vi "data insert core.vi"(8 "error in (no error)":errorcluster, 9 "column information":T1[](array[typedef]), 10 "data":variant[](array[variant]), 11 "table":string) -> (0 "error out":errorcluster)   [LabVIEW 2016, in "质控单元.lvlib"]
uses:
  <vilib>/addons/database/Auxilliary.llb/DB Tools Column Info.ctl
  <vilib>/addons/database/Auxilliary.llb/DB Tools DataTypes.ctl
  <vilib>/addons/database/Auxilliary.llb/DB Tools Transaction.ctl
  <vilib>/addons/database/Auxilliary.llb/DB Tools Isolation Level.ctl
  <vilib>/Utility/sysdir.llb/System Directory Type.ctl
  <vilib>/addons/database/Auxilliary.llb/DB Tools Parameter Info.ctl
  <vilib>/addons/database/Auxilliary.llb/DB Tools Parameter Dir.ctl
  <vilib>/addons/database/Connection.llb/DB Tools Open Connec (String).vi
  <vilib>/addons/database/Connection.llb/Conn Transaction.vi
  <vilib>/addons/database/Connection.llb/Conn Execute.vi
  <vilib>/addons/database/Recordset.llb/Rec Destroy - Connection.vi
  <vilib>/addons/database/Command.llb/Cmd Set Parameter Value (C).vi
  <vilib>/addons/database/Auxilliary.llb/DB Tools Format Datetime String (Time Stamp).vi
  <vilib>/addons/database/Command.llb/Cmd Execute.vi
  <vilib>/addons/database/Recordset.llb/Rec Destroy - Command.vi
  <vilib>/addons/database/Command.llb/Cmd Delete.vi
  <vilib>/addons/database/NI_Database_API.lvlib
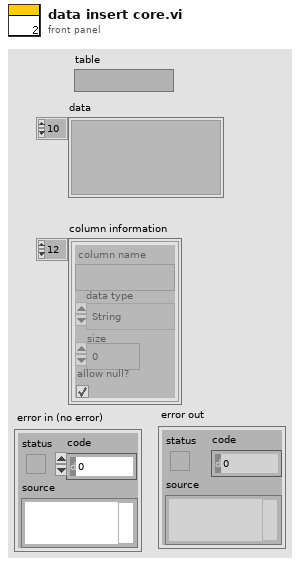
[diagram p1: front panel]
types:
  T1 = typedef "NI_Database_API.lvlib/DB Tools Column Info.ctl" = cluster{"column name":string, "data type":T2, "size":i32, "allow null?":bool}
  T2 = typedef "NI_Database_API.lvlib/DB Tools DataTypes.ctl" = enum16{"String", "Long (I32)", "Single (SGL)", "Double (DBL)", "Date/Time", "Binary"}
  T3 = typedef "System Directory Type.ctl" = i32
  T4 = typedef "NI_Database_API.lvlib/DB Tools Isolation Level.ctl" = enum16{"chaos", "read uncommitted", "read committed", "repeatable read", "serializable"}
  T5 = typedef "NI_Database_API.lvlib/DB Tools Transaction.ctl" = enum16{"begin", "commit", "rollback"}
  T6 = typedef "NI_Database_API.lvlib/Conn ObjectReference.ctl" = refnum<k1>
  T7 = typedef "NI_Database_API.lvlib/DB Tools Parameter Info.ctl" = cluster{"parameter name":string, "type":T2, "direction":T8, "value":variant}
  T8 = typedef "NI_Database_API.lvlib/DB Tools Parameter Dir.ctl" = enum32{"Input", "Output", "Input/Output", "Return Value"}
  T9 = typedef "NI_Database_API.lvlib/Rec ObjectReference.ctl" = refnum<k1>
  T10 = typedef "NI_Database_API.lvlib/Cmd ObjectReference.ctl" = refnum<k1>
  T11 = typedef "NI_Database_API.lvlib/Cmd-Rec Object Reference.ctl" = refnum<k1>
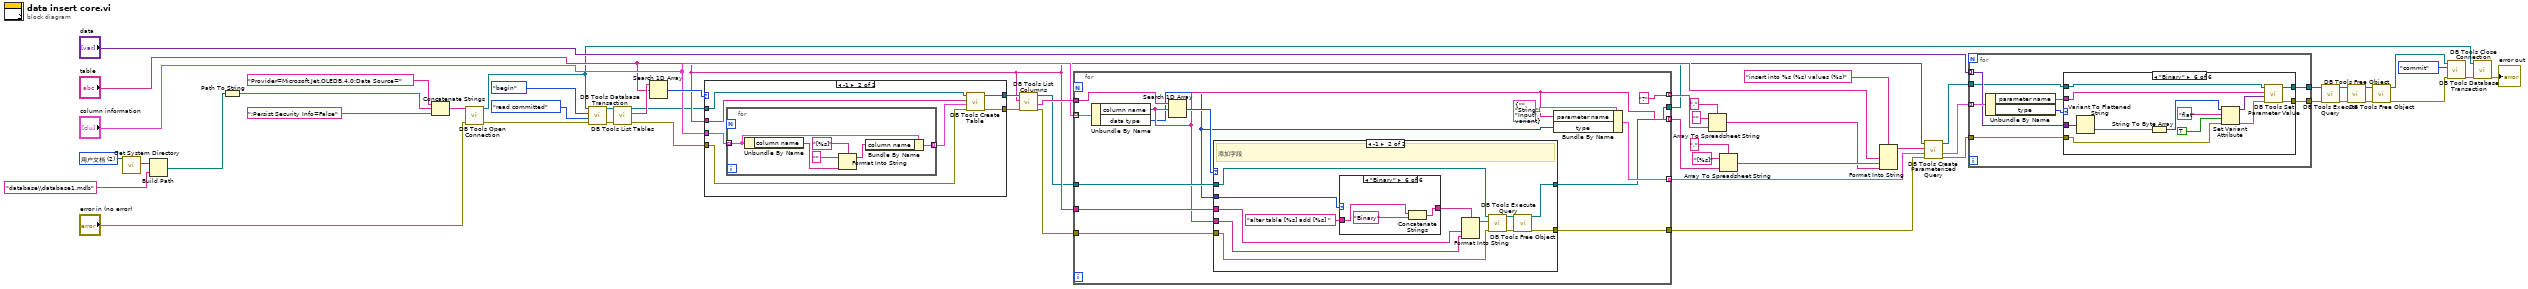
[diagram p0: block diagram]
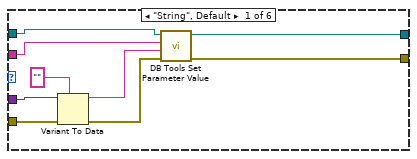
[diagram p2: hidden frame]
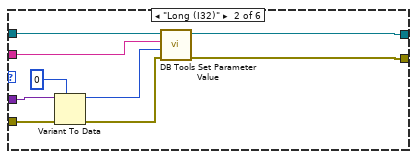
[diagram p3: hidden frame]
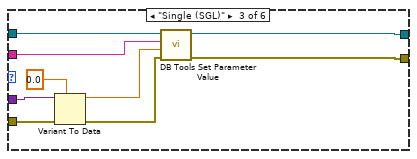
[diagram p4: hidden frame]
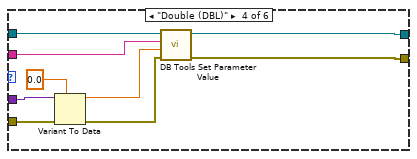
[diagram p5: hidden frame]
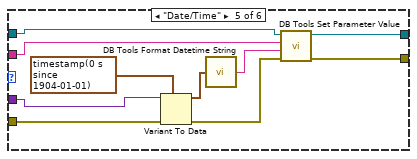
[diagram p6: hidden frame]
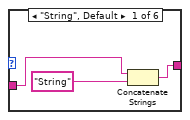
[diagram p8: hidden frame]
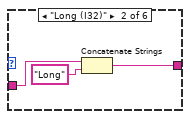
[diagram p9: hidden frame]
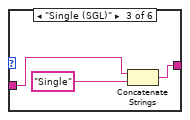
[diagram p10: hidden frame]
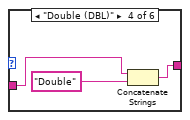
[diagram p11: hidden frame]
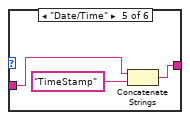
[diagram p12: hidden frame]
diagram:
  w3 = T3 2 items=["用户目录"=0, "用户桌面"=1, "用户文档"=2, "用户应用程序数据"=3, "用户设置"=4, "用户临时目录"=5, "公共文档"=6, "公共应用程序数据"=7, "公共设置"=8, "公共缓存"=13, "系统核心库"=9, "系统安装库"=10, "应用程序文件"=11, "启动盘根目录"=12] ("system directory type")
  n1 = call <vilib>:"Get System Directory.vi"("system directory type"=w3) -> ("system directory"=w4:path)  [unwired: 10 in]
  n2 = Build Path(base path=w4, name or relative path="database\\database1.mdb" ("名称或相对路径")) -> (appended path=w2:path)
  n3 = Path To String(path=w2) -> (string=w53:string)
  n4 = Concatenate Strings("Provider=Microsoft.Jet.OLEDB.4.0;Data Source=" ("condition"), w53, ";Persist Security Info=False" ("condition")) -> (w51:string)
  n5 = call-poly <vilib>:"DB Tools Open Connection.vi"("error in (no error)"="error in (no error)", "connection information"=w51) -> ("error out"=w13:errorcluster, "connection reference"=w5:T6)  [unwired: 6 in]
  n6 = call-poly <vilib>:"DB Tools Database Transaction.vi"("error in (no error)"=w13, "isolation level (chaos)"=DB_Tools_Isolation_Level."read committed", "operation (begin)"=DB_Tools_Transaction."begin", "connection reference"=w5) -> ("error out"=w12:errorcluster, "connection reference out"=w14:T6)  [unwired: 2 in]
  n7 = call <vilib>:"DB Tools List Tables.vi"("error in (no error)"=w12, "connection reference"=w14) -> ("error out"=w43:errorcluster, "tables"=w45:string[], "connection reference out"=w8:T6)  [unwired: 3 in]
  n8 = Search 1D Array(1D array=w45, element="table") -> (index of element=w44:i32)  [unwired: 1 in]
  n9 = case shown="-1" w44 {
    tunnel: w8 -> [w56 w63]
    tunnel: w43 -> [w55 w62]
    tunnel: "table" -> [_ w61]
    tunnel: "column information" -> [_ w58]
    tunnel: [w56 w60] -> w39
    tunnel: [w55 w59] -> w38
    frame 0, Default {
    }
    frame -1 {
      n10 = for {
        tunnel: w58 -> [w65] mode=indexing
        tunnel: [w64] -> w57 mode=indexing
        n11 = Unbundle By Name(w65) -> ("column name"=w69:string)
        n12 = Format Into String(format string="[%s]" ("格式字符串"), initial string="" ("初始字符串"), w69) -> (resulting string=w66:string)  [unwired: 1 in, 1 out]
        n13 = Bundle By Name(cluster=w65, "column name"=w66) -> (w64:T1)
      }
      n14 = call <vilib>:"DB Tools Create Table.vi"("error in (no error)"=w62, "column information"=w57, "table"=w61, "connection reference"=w63) -> ("error out"=w59:errorcluster, "connection reference out"=w60:T6)  [unwired: 4 in]
    }
  }
  n15 = call <vilib>:"DB Tools List Columns.vi"("error in (no error)"=w38, "table"="table", "connection reference"=w39) -> ("error out"=w41:errorcluster, "columns"=w42:string[], "connection reference out"=w10:T6)  [unwired: 1 in, 1 out]
  n16 = for {
    tunnel: w10 -> [w80]
    tunnel: w42 -> [w82]
    tunnel: w41 -> [w79]
    tunnel: [w78] -> w37
    tunnel: "table" -> [w77]
    tunnel: "column information" -> [w76] mode=indexing
    tunnel: [w74] -> w36 mode=indexing
    tunnel: [w73] -> w29 mode=indexing
    tunnel: ["?"] -> w27 mode=indexing
    tunnel: [w70] -> w7
    n17 = Unbundle By Name(w76) -> ("column name"=w73:string, "data type"=w71:T2)
    n18 = Search 1D Array(1D array=w82, element=w73) -> (index of element=w81:i32)  [unwired: 1 in]
    n19 = case shown="-1" w81 {
      tunnel: [w84 w93] -> w78
      tunnel: w80 -> [w83 w92]
      tunnel: w73 -> [_ w91]
      tunnel: w79 -> [w84 w90]
      tunnel: w77 -> [_ w89]
      tunnel: w71 -> [_ w87]
      tunnel: [w83 w85] -> w70
      frame 0, Default {
      }
      frame -1 {
        # "添加字段"
        n20 = case shown="\"Binary\"" w87 {
          tunnel: "alter table [%s] add [%s] " -> [w99 w102 w105 w108 w111 w114]
          tunnel: [w98 w101 w104 w107 w110 w113] -> w86
          frame "String", Default {
            n21 = Concatenate Strings(w99, "String" ("字符串")) -> (w98:string)
          }
          frame "Long (I32)" {
            n22 = Concatenate Strings(w102, "Long" ("字符串")) -> (w101:string)
          }
          frame "Single (SGL)" {
            n23 = Concatenate Strings(w105, "Single" ("字符串")) -> (w104:string)
          }
          frame "Double (DBL)" {
            n24 = Concatenate Strings(w108, "Double" ("字符串")) -> (w107:string)
          }
          frame "Date/Time" {
            n25 = Concatenate Strings(w111, "TimeStamp" ("字符串")) -> (w110:string)
          }
          frame "Binary" {
            n26 = Concatenate Strings(w114, "Binary" ("字符串")) -> (w113:string)
          }
        }
        n27 = Format Into String(format string=w86, w89, w91) -> (resulting string=w94:string)  [unwired: 2 in, 1 out]
        n28 = call-poly <vilib>:"DB Tools Execute Query.vi"("error in (no error)"=w90, "SQL query"=w94, "connection reference"=w92) -> ("error out"=w95:errorcluster, "recordset reference"=w96:T9)  [unwired: 5 in]
        n29 = call-poly <vilib>:"DB Tools Free Object.vi"("error in (no error)"=w95, "recordset reference"=w96) -> ("error out"=w93:errorcluster, "connection reference"=w85:T6)  [unwired: 8 in]
      }
    }
    n30 = Bundle By Name(cluster=T7 {"parameter name"="", "type"=enum."String", "direction"=enum."Input", "value"=variant} ("parameter information"), "parameter name"=w73, "type"=w71) -> (w74:T7)
  }
  n31 = Array To Spreadsheet String(delimiter (Tab)="," ("分隔符(Tab)"), array=w27, 3:"" ("格式字符串")) -> (spreadsheet string=w26:string)
  n32 = Array To Spreadsheet String(delimiter (Tab)="," ("分隔符(Tab)"), array=w29, 3:"[%s]" ("格式字符串")) -> (spreadsheet string=w28:string)
  n33 = Format Into String(format string="insert into %s (%s) values (%s)" ("格式字符串"), "table", w28, w26) -> (resulting string=w25:string)  [unwired: 2 in, 1 out]
  n34 = call <vilib>:"DB Tools Create Parameterized Query.vi"("error in (no error)"=w37, "parameters"=w36, "SQL query"=w25, "connection reference"=w7) -> ("error out"=w24:errorcluster, "parameters out"=w23:T7[], "command reference"=w9:T10)  [unwired: 3 in]
  n35 = for {
    tunnel: w9 -> [w119]
    tunnel: w24 -> [w117]
    tunnel: w23 -> [w122] mode=indexing
    tunnel: "data" -> [w120] mode=indexing
    tunnel: [w116] -> w6
    tunnel: [w115] -> w22
    n36 = Unbundle By Name(w122) -> ("parameter name"=w118:string, "type"=w121:T2)
    n37 = case shown="\"Binary\"" w121 {
      tunnel: w120 -> [w126 w134 w141 w151 w168 w172]
      tunnel: w119 -> [w129 w138 w145 w155 w166 w180]
      tunnel: w118 -> [w128 w137 w144 w150 w165 w179]
      tunnel: w117 -> [w123 w132 w142 w152 w163 w171]
      tunnel: [w125 w136 w146 w154 w162 w178] -> w116
      tunnel: [w124 w135 w143 w153 w161 w177] -> w115
      frame "String", Default {
        n38 = Variant To Data(error in=w123, type="", Variant=w126) -> (data=w127:string, error out=w131:errorcluster)
        n39 = call-poly <vilib>:"DB Tools Set Parameter Value.vi"("error in (no error)"=w131, "value"=w127, "parameter index"=w128, "command reference"=w129) -> ("error out"=w124:errorcluster, "command reference out"=w125:T10)  [unwired: 4 in]
      }
      frame "Long (I32)" {
        n40 = Variant To Data(error in=w132, type=0, Variant=w134) -> (data=w139:i32, error out=w140:errorcluster)
        n41 = call-poly <vilib>:"DB Tools Set Parameter Value.vi"("error in (no error)"=w140, "value"=w139, "parameter index"=w137, "command reference"=w138) -> ("error out"=w135:errorcluster, "command reference out"=w136:T10)  [unwired: 4 in]
      }
      frame "Single (SGL)" {
        n42 = Variant To Data(error in=w142, type=sgl 0.0, Variant=w141) -> (data=w148:sgl, error out=w149:errorcluster)
        n43 = call-poly <vilib>:"DB Tools Set Parameter Value.vi"("error in (no error)"=w149, "value"=w148, "parameter index"=w144, "command reference"=w145) -> ("error out"=w143:errorcluster, "command reference out"=w146:T10)  [unwired: 4 in]
      }
      frame "Double (DBL)" {
        n44 = Variant To Data(error in=w152, type=0.0, Variant=w151) -> (data=w157:dbl, error out=w158:errorcluster)
        n45 = call-poly <vilib>:"DB Tools Set Parameter Value.vi"("error in (no error)"=w158, "value"=w157, "parameter index"=w150, "command reference"=w155) -> ("error out"=w153:errorcluster, "command reference out"=w154:T10)  [unwired: 4 in]
      }
      frame "Date/Time" {
        n46 = Variant To Data(error in=w163, type=timestamp(0 s since 1904-01-01) ("时间标识"), Variant=w168) -> (data=w160:timestamp, error out=w164:errorcluster)
        n47 = call-poly <vilib>:"DB Tools Format Datetime String.vi"("time stamp"=w160) -> ("date/time string"=w159:string)
        n48 = call-poly <vilib>:"DB Tools Set Parameter Value.vi"("error in (no error)"=w164, "value"=w159, "parameter index"=w165, "command reference"=w166) -> ("error out"=w161:errorcluster, "command reference out"=w162:T10)  [unwired: 4 in]
      }
      frame "Binary" {
        n49 = Variant To Flattened String(Variant=w172) -> (data string=w173:string)  [unwired: 1 out]
        n50 = String To Byte Array(string=w173) -> (unsigned byte array=w176:u8[])
        n51 = Set Variant Attribute(Variant=w176, name="flat", value=TRUE, error in=w171) -> (Variant out=w169:variant, error out=w170:errorcluster)  [unwired: 1 out]
        n52 = call-poly <vilib>:"DB Tools Set Parameter Value.vi"("error in (no error)"=w170, "value"=w169, "parameter index"=w179, "command reference"=w180) -> ("error out"=w177:errorcluster, "command reference out"=w178:T10)  [unwired: 4 in]
      }
    }
  }
  n53 = call-poly <vilib>:"DB Tools Execute Query.vi"("error in (no error)"=w22, "command reference"=w6) -> ("error out"=w20:errorcluster, "command-recordset reference"=w21:T11)  [unwired: 6 in]
  n54 = call-poly <vilib>:"DB Tools Free Object.vi"("error in (no error)"=w20, "command-recordset reference"=w21) -> ("error out"=w18:errorcluster, "command reference"=w19:T10)  [unwired: 8 in]
  n55 = call-poly <vilib>:"DB Tools Free Object.vi"("error in (no error)"=w18, "command reference"=w19) -> ("error out"=w15:errorcluster, "connection reference"=w16:T6)  [unwired: 8 in]
  n56 = call-poly <vilib>:"DB Tools Database Transaction.vi"("error in (no error)"=w15, "operation (begin)"=DB_Tools_Transaction."commit", "connection reference"=w16) -> ("error out"=w17:errorcluster)  [unwired: 3 in, 1 out]
  n57 = call <vilib>:"DB Tools Close Connection.vi"("error in (no error)"=w17, "connection reference"=w5) -> ("error out"=→"error out":errorcluster)  [unwired: 5 in]
